vi "YAV_90132_RESET_TS.vi"(1 "Address":u8, 3 "error in (no error)":errorcluster) -> (5 "error out":errorcluster)   [LabVIEW 2018]
uses:
  <instrlib>/Phi6/Common/Instrum/Phi6 Core/YAV-System.llb/YAV Card Total Info.ctl
  <instrlib>/Phi6/Common/Instrum/Phi6 Core/YAV-System.llb/YAV Info.ctl
  <instrlib>/Phi6/Common/Instrum/Phi6 Core/YAV-90132.llb/YAV90132 Mode Action.ctl
  <instrlib>/Phi6/Common/Instrum/Phi6 Core/YAV-90132.llb/YAV90132 Type Action.ctl
  <instrlib>/Phi6/Common/Instrum/Phi6 Core/CANNOU Global Variables.llb/CANNOU Global Variables.gbl.vi
panel:
  in  "Info In":T1 {"Version" format="%.0x"; "Options" format="%.0x"; "Index" format="%.0x"}
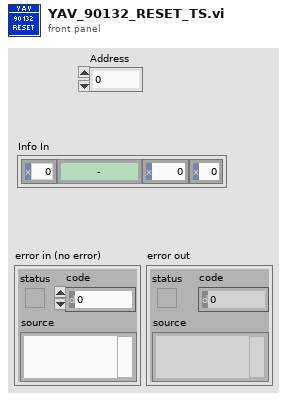
[diagram p1: front panel]
types:
  T1 = typedef "YAV Card Total Info.ctl" = cluster{"Index":u8, "Module":T2, "Version":u16, "Options":u8}
  T2 = typedef "YAV Info.ctl" = enum16{"-", "YAV90832", "YAV904X8", "YAV90132", "YAV91616", "YAV90PIN", "YAV90096", "YAV90HVT", "YAV90CLR", "YAV90128", "YAV90PNE", "YAVCANCON", "YAV91775", "YAV90XXX", "YAV90MMU", "H730050", "H710060", "H710061", "YAV90304", "MMI", "YAV90060", "YAV90MUX", "YAV90059", "YAV90070", "AK087", "Not Defined"}
  T3 = typedef "Module CAN.ctl" = enum16{"CAN0", "CAN1", "CAN2", "CAN3", "CAN4", "CAN5"}
  T4 = typedef "YAV90132 Type Action.ctl" = enum16{"None", "Set OFF", "Set ON", "TOGGLE", "BLINK", "PULSE ON", "PULSE OFF", "ASK", "Set OUT"}
  T5 = typedef "YAV90132 Mode Action.ctl" = enum16{"None", "One Relay", "Several Relays"}
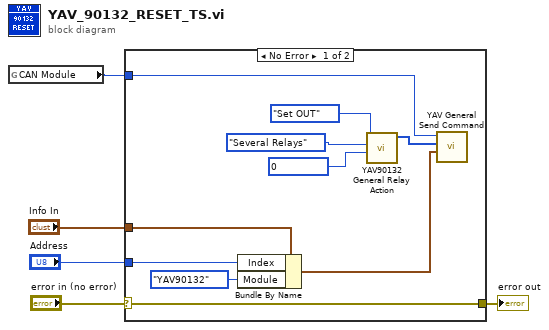
[diagram p0: block diagram]
diagram:
  n1 = global read "CANNOU Global Variables.gbl.vi" "CAN Module"() -> (w1:T3)
  n2 = case shown="No Error" "error in (no error)" {
    selector: "error in (no error)" -> [w8 w16]
    tunnel: w1 -> [w15 _]
    tunnel: "Info In" -> [w12 _]
    tunnel: "Address" -> [w9 _]
    tunnel: [w8 w16] -> w2
    frame No Error {
      n3 = Bundle By Name(cluster=w12, "Index"=w9, "Module"=YAV_Info."YAV90132") -> (w11:T1)
      n4 = call <instrlib>:"YAV90132 General Relay Action.vi"("Relay/Relays"=u32 0, "Mode Action"=YAV90132_Mode_Action."Several Relays", "Type Action"=YAV90132_Type_Action."Set OUT") -> ("Data"=w14:u8[])  [unwired: 8 in]
      n5 = call <instrlib>:"YAV General Send Command.vi"("Info In"=w11, "Data"=w14, "CAN Module"=w15) -> ()  [unwired: 3 in, 2 out]
    }
    frame Error {
    }
  }
  "error out" <- w2
